vi "Copy_with_Check.vi"(1 "Mode":enum16{"Move", "Copy"}(ring)=enum."Copy", 2 "Target Path":path, 3 "Variable Target?":bool, 4 "Source Path":path) -> (0 "Pathname Out":path)   [LabVIEW 2010]
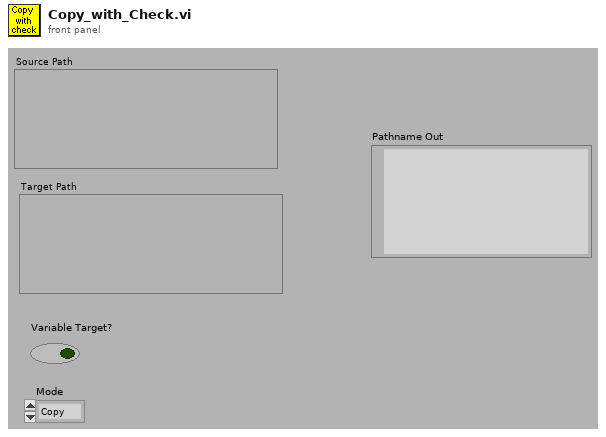
[diagram p1: front panel]
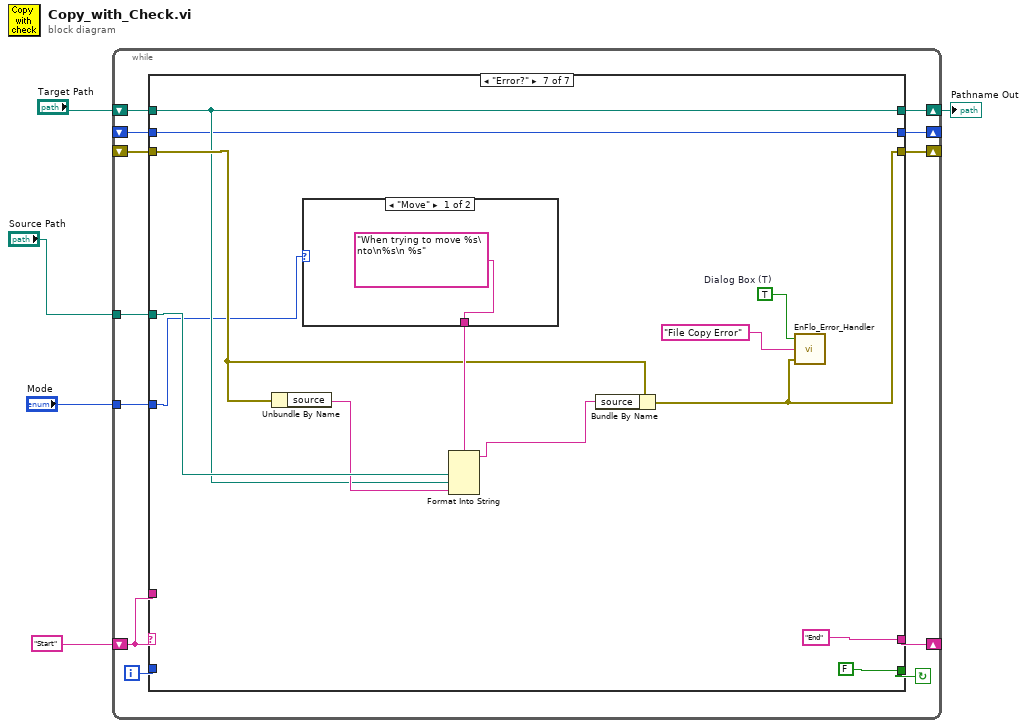
[diagram p0: block diagram]
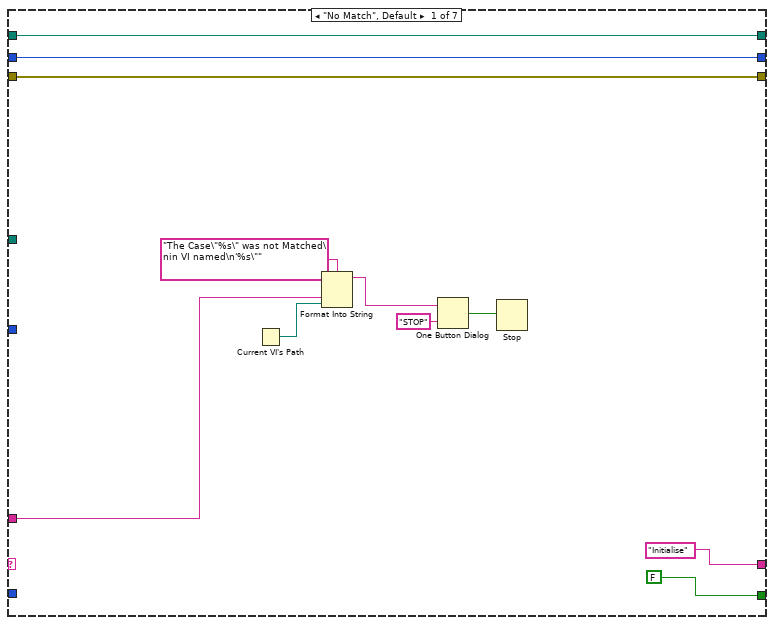
[diagram p2: hidden frame]
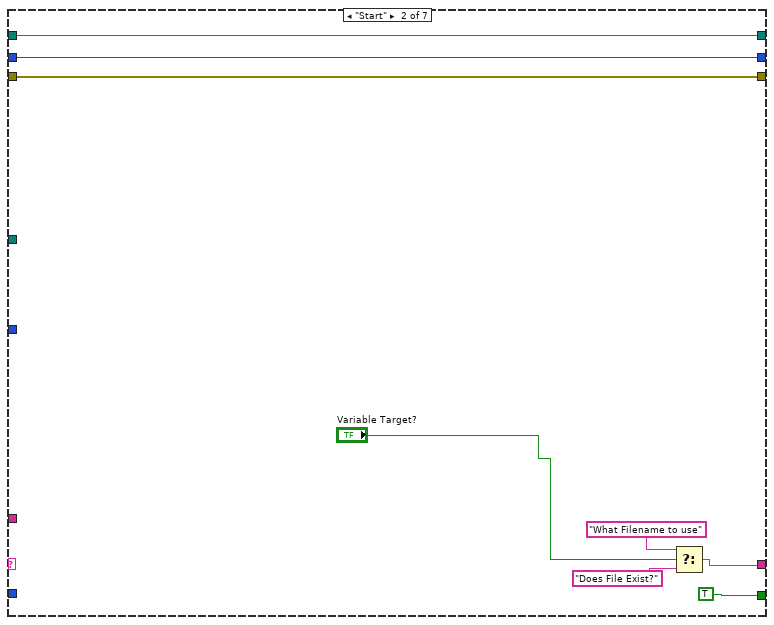
[diagram p3: hidden frame]
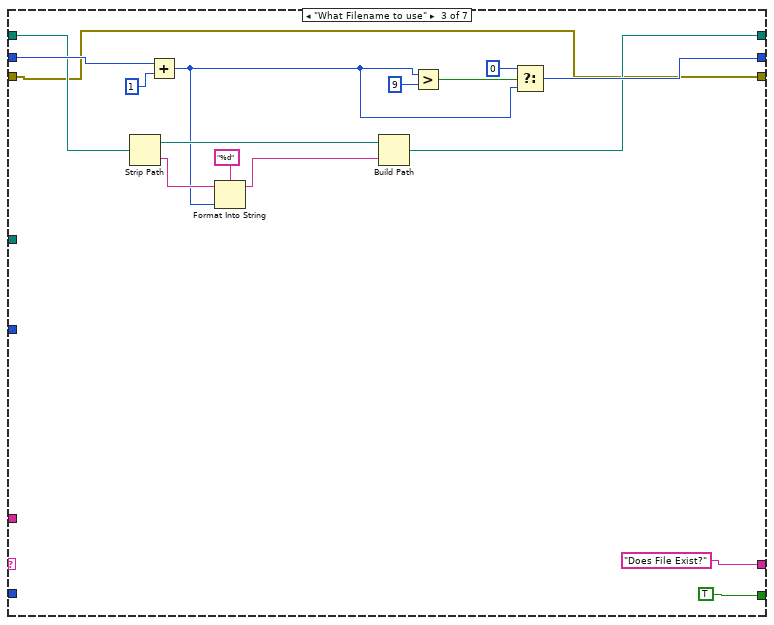
[diagram p4: hidden frame]
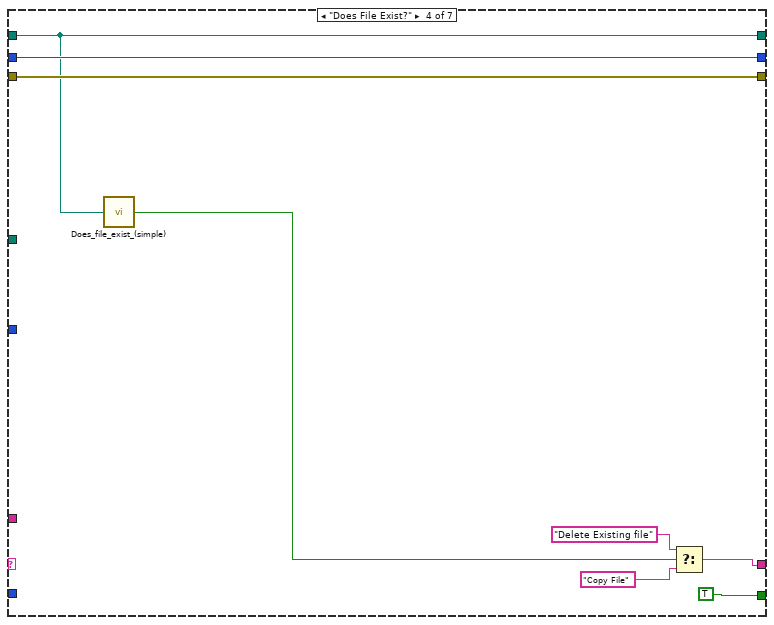
[diagram p5: hidden frame]
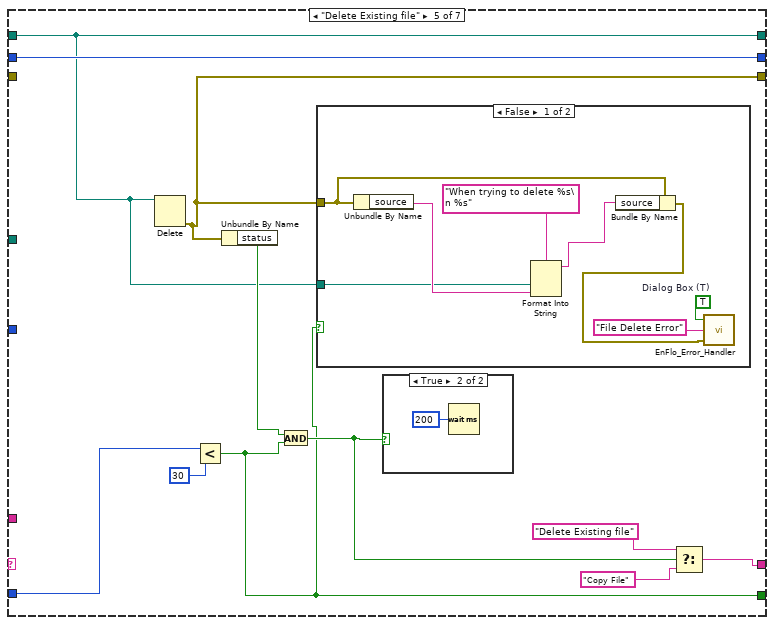
[diagram p6: hidden frame]
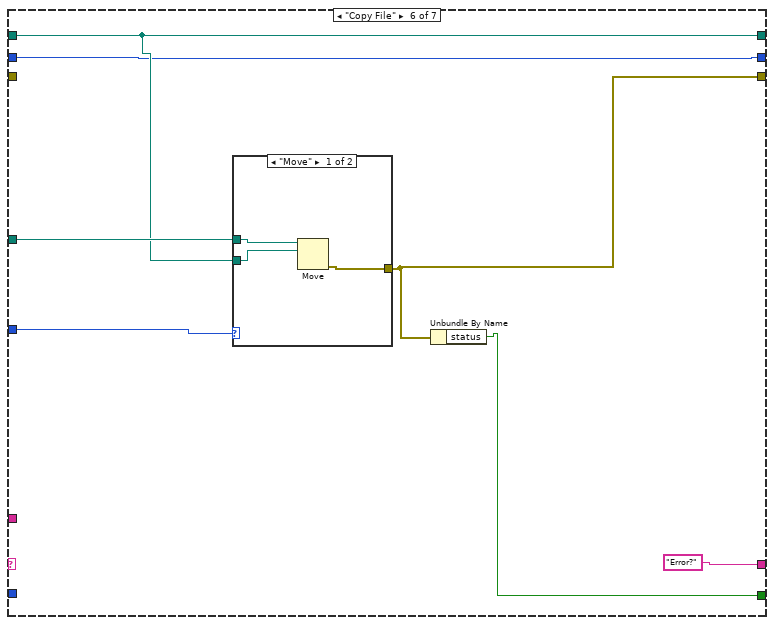
[diagram p9: hidden frame]
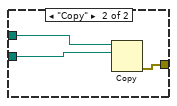
[diagram p10: hidden frame]
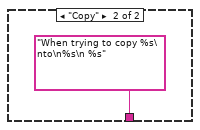
[diagram p11: hidden frame]
diagram:
  n1 = while {
    shift-left: "Start" -> [w15]
    shift-right: [w16] -> _
    shift-right: [w11] -> w3
    shift-left: "Target Path" -> [w14]
    shift-right: [w12] -> _
    shift-left: _ -> [w13]
    shift-right: [w10] -> _
    shift-left: _ -> [w9]
    tunnel: "Source Path" -> [w8]
    tunnel: "Mode" -> [w6]
    i -> [w7]
    stop <- w17 continue-if-true
    n2 = case shown="\"Error?\"" w15 {
      tunnel: [FALSE TRUE TRUE TRUE w63 w85 FALSE] -> w17
      tunnel: ["Initialise" w33 "Does File Exist?" ("f") w58 w71 "Error?" "End"] -> w16
      tunnel: w15 -> [w23 _ _ _ _ _ _]
      tunnel: w14 -> [w20 w35 w49 w54 w61 w83 w97]
      tunnel: w13 -> [w19 w30 w51 w55 w69 w82 w96]
      tunnel: [w19 w30 w40 w55 w69 w82 w96] -> w12
      tunnel: [w20 w35 w39 w54 w61 w83 w97] -> w11
      tunnel: [w18 w29 w37 w56 w62 w86 w95] -> w10
      tunnel: w9 -> [w18 w29 w37 w56 _ _ w99]
      tunnel: w8 -> [_ _ _ _ _ w84 w102]
      tunnel: w7 -> [_ _ _ _ w67 _ _]
      tunnel: w6 -> [_ _ _ _ _ w81 w94]
      frame "No Match", Default {
        n3 = Current VI's Path() -> (path=w22:path)
        n4 = Format Into String(format string="The Case\"%s\" was not Matched\nin VI named\n'%s\"" ("Format String"), w23, w22) -> (resulting string=w26:string)  [unwired: 2 in, 1 out]
        n5 = One Button Dialog(message=w26, button name ("OK")="STOP") -> (true=w24:bool)
        n6 = Stop(stop? (T)=w24) -> ()
      }
      frame "Start" {
        n7 = Select(t="What Filename to use", s="Variable Target?", f="Does File Exist?") -> (s? t:f=w33:string)
      }
      frame "What Filename to use" {
        n8 = Strip Path(path=w49) -> (stripped path=w46:path, name=w48:string)
        n9 = Add(x=w51, y=1) -> (x+y=w42:i32)
        n10 = Format Into String(format string="%d", initial string=w48, w42) -> (resulting string=w45:string)  [unwired: 1 in, 1 out]
        n11 = Build Path(base path=w46, name or relative path=w45) -> (appended path=w39:path)
        n12 = Greater?(x=w42, y=9) -> (0:w43:bool)
        n13 = Select(t=0, s=w43, f=w42) -> (s? t:f=w40:i32)
      }
      frame "Does File Exist?" {
        n14 = call "Does_file_exist_(simple).vi"("Pathname"=w54) -> ("exists?"=w59:bool)
        n15 = Select(t="Delete Existing file", s=w59, f="Copy File") -> (s? t:f=w58:string)
      }
      frame "Delete Existing file" {
        n16 = Delete(path (use dialog)=w61) -> (error out=w62:errorcluster)  [unwired: 1 in, 5 out]
        n17 = Less?(x=w67, y=30) -> (x < y?=w63:bool)
        n18 = Unbundle By Name(w62) -> ("status"=w66:bool)
        n19 = And(x=w66, y=w63) -> (x .and. y?=w65:bool)
        n20 = case shown="False" w63 {
          tunnel: w62 -> [w75 _]
          tunnel: w61 -> [w76 _]
          frame False {
            w74 = TRUE  # Dialog Box (T)
            n21 = Unbundle By Name(w75) -> ("source"=w79:string)
            n22 = Format Into String(format string="When trying to delete %s\n %s", w76, w79) -> (resulting string=w77:string)  [unwired: 2 in, 1 out]
            n23 = Bundle By Name(cluster=w75, "source"=w77) -> (w72:errorcluster)
            n24 = call "EnFlo_Error_Handler.vi"("error in (no error)"=w72, "Error Type"="File Delete Error", "Dialog Box (T)"=w74) -> ()  [unwired: 3 out]
          }
          frame True {
          }
        }
        n25 = case shown="True" w65 {
          frame False {
          }
          frame True {
            n26 = Wait (ms)(milliseconds to wait=u32 200) -> ()  [unwired: 1 out]
          }
        }
        n27 = Select(t="Delete Existing file", s=w65, f="Copy File") -> (s? t:f=w71:string)
      }
      frame "Copy File" {
        n28 = case shown="\"Move\"" w81 {
          tunnel: [w88 w93] -> w86
          tunnel: w84 -> [w90 w92]
          tunnel: w83 -> [w89 w91]
          frame "Move" {
            n29 = Move(source path=w90, 10:w89) -> (error out=w88:errorcluster)  [unwired: 1 in, 4 out]
          }
          frame "Copy" {
            n30 = Copy(10:w91, 11:w92) -> (0:w93:errorcluster)  [unwired: 1 in, 4 out]
          }
        }
        n31 = Unbundle By Name(w86) -> ("status"=w85:bool)
      }
      frame "Error?" {
        w104 = TRUE  # Dialog Box (T)
        n32 = Unbundle By Name(w99) -> ("source"=w101:string)
        n33 = case shown="\"Move\"" w94 {
          tunnel: ["When trying to move %s\nto\n%s\n %s" ("format string") "When trying to copy %s\nto\n%s\n %s" ("format string")] -> w100
          frame "Move" {
          }
          frame "Copy" {
          }
        }
        n34 = Format Into String(format string=w100, w102, w97, w101) -> (resulting string=w98:string)  [unwired: 2 in, 1 out]
        n35 = Bundle By Name(cluster=w99, "source"=w98) -> (w95:errorcluster)
        n36 = call "EnFlo_Error_Handler.vi"("error in (no error)"=w95, "Error Type"="File Copy Error", "Dialog Box (T)"=w104) -> ()  [unwired: 3 out]
      }
    }
  }
  "Pathname Out" <- w3
